vi "pH电极校准.vi"() -> ()   [LabVIEW 2016, in "斯坦道多参数.lvlib"]
uses:
  <vilib>/Utility/miscctls.llb/LVPointTypeDef.ctl
  <vilib>/Analysis/NI_AALBase.lvlib
panel:
  in  "校准停止":bool
  in  "校准启动":bool
  out "第二点校准值":dbl
  out "第一点校准值":dbl
  out "提示":string
  in  "校准模式":enum16{"两点校准", "单点校准"}(ring)
  out "最小值":sgl format="%.2g"
  out "最大值":sgl format="%.2g"
  out "变异系数":dbl format="%.6g"
  out "standard deviation":dbl caption="标准差" format="%0.2f"
  out "mean":dbl caption="均值" format="%0.2f"
  out "波形图表":sgl(graph) caption="历史曲线"
  out "当前检测值":dbl format="%#.2g"
  out "标液2":dbl
  out "标液1":dbl
  out "当前信号值":dbl format="%#.2g"
  out "偏移值补偿":dbl format="%#.2g"
  out "电极斜率":dbl
  out "电极零点":dbl
  # "酸碱度电极设定"
  # "mV"
  # "mV"
  # "%"
  # "pH"
  # "请选择校准模式:"
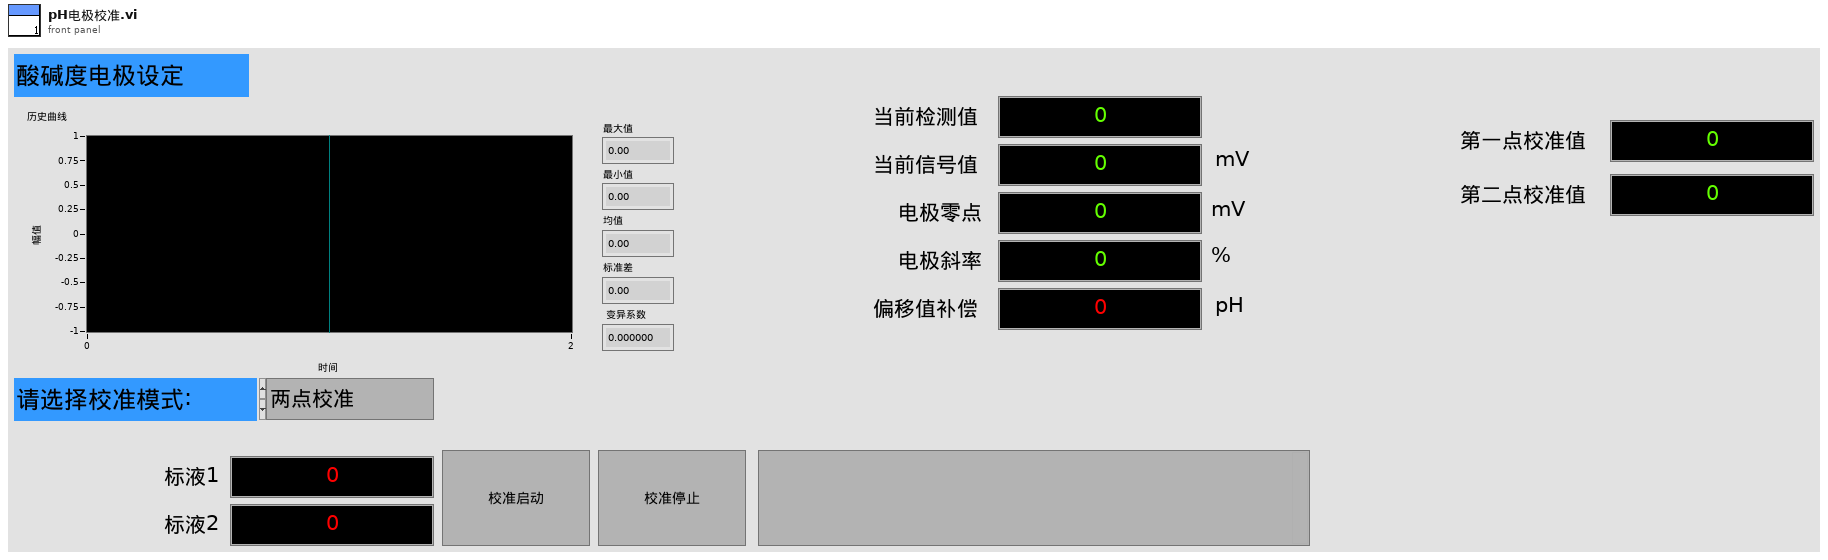
[diagram p1: front panel]
types:
  T1 = typedef "LVPointTypeDef.ctl" = cluster{"Horizontal":i16, "Vertical":i16}
  T2 = typedef "斯坦道多参数.lvlib/校准步骤.ctl" = enum16{"待机", "放置第一点标液", "第一点校准启动", "第一点校准写入", "第一点校准失败", "放置第二点标液", "第二点校准启动", "第二点校准写入", "第二点校准失败", "校准结果写入", "校准结束"}
  T3 = cluster{"电极状态标志":u16, "电极型号标志":u16, "酸碱度测量值":sgl, "温度测量值":sgl, "酸碱度信号值":sgl, "温度信号值":sgl, "酸碱度偏移修正值":sgl, "温度偏移修正值":sgl, "手动温度补偿值":sgl, "酸碱度电极零点":sgl, "酸碱度电极斜率":sgl, "第1点标准值记录":sgl, "第1点信号值记录":sgl, "第1点温度值记录":sgl, "第2点标准值记录":sgl, "第2点信号值记录":sgl, "第2点温度值记录":sgl, "命令滤波设定":u16, "温度模式":enum16{"ATC", "MTC"}, "生产批次":u16, "电极序号":u16, "串口地址":u16, "串口波特率":enum16{"9600", "19200", "115200"}, "串口校验位":enum16{"NONE", "ODD", "EVEN"}, "串口停止位":enum16{"1bit", "2bit"}, "第一点标准值":sgl, "第二点标准值":sgl}
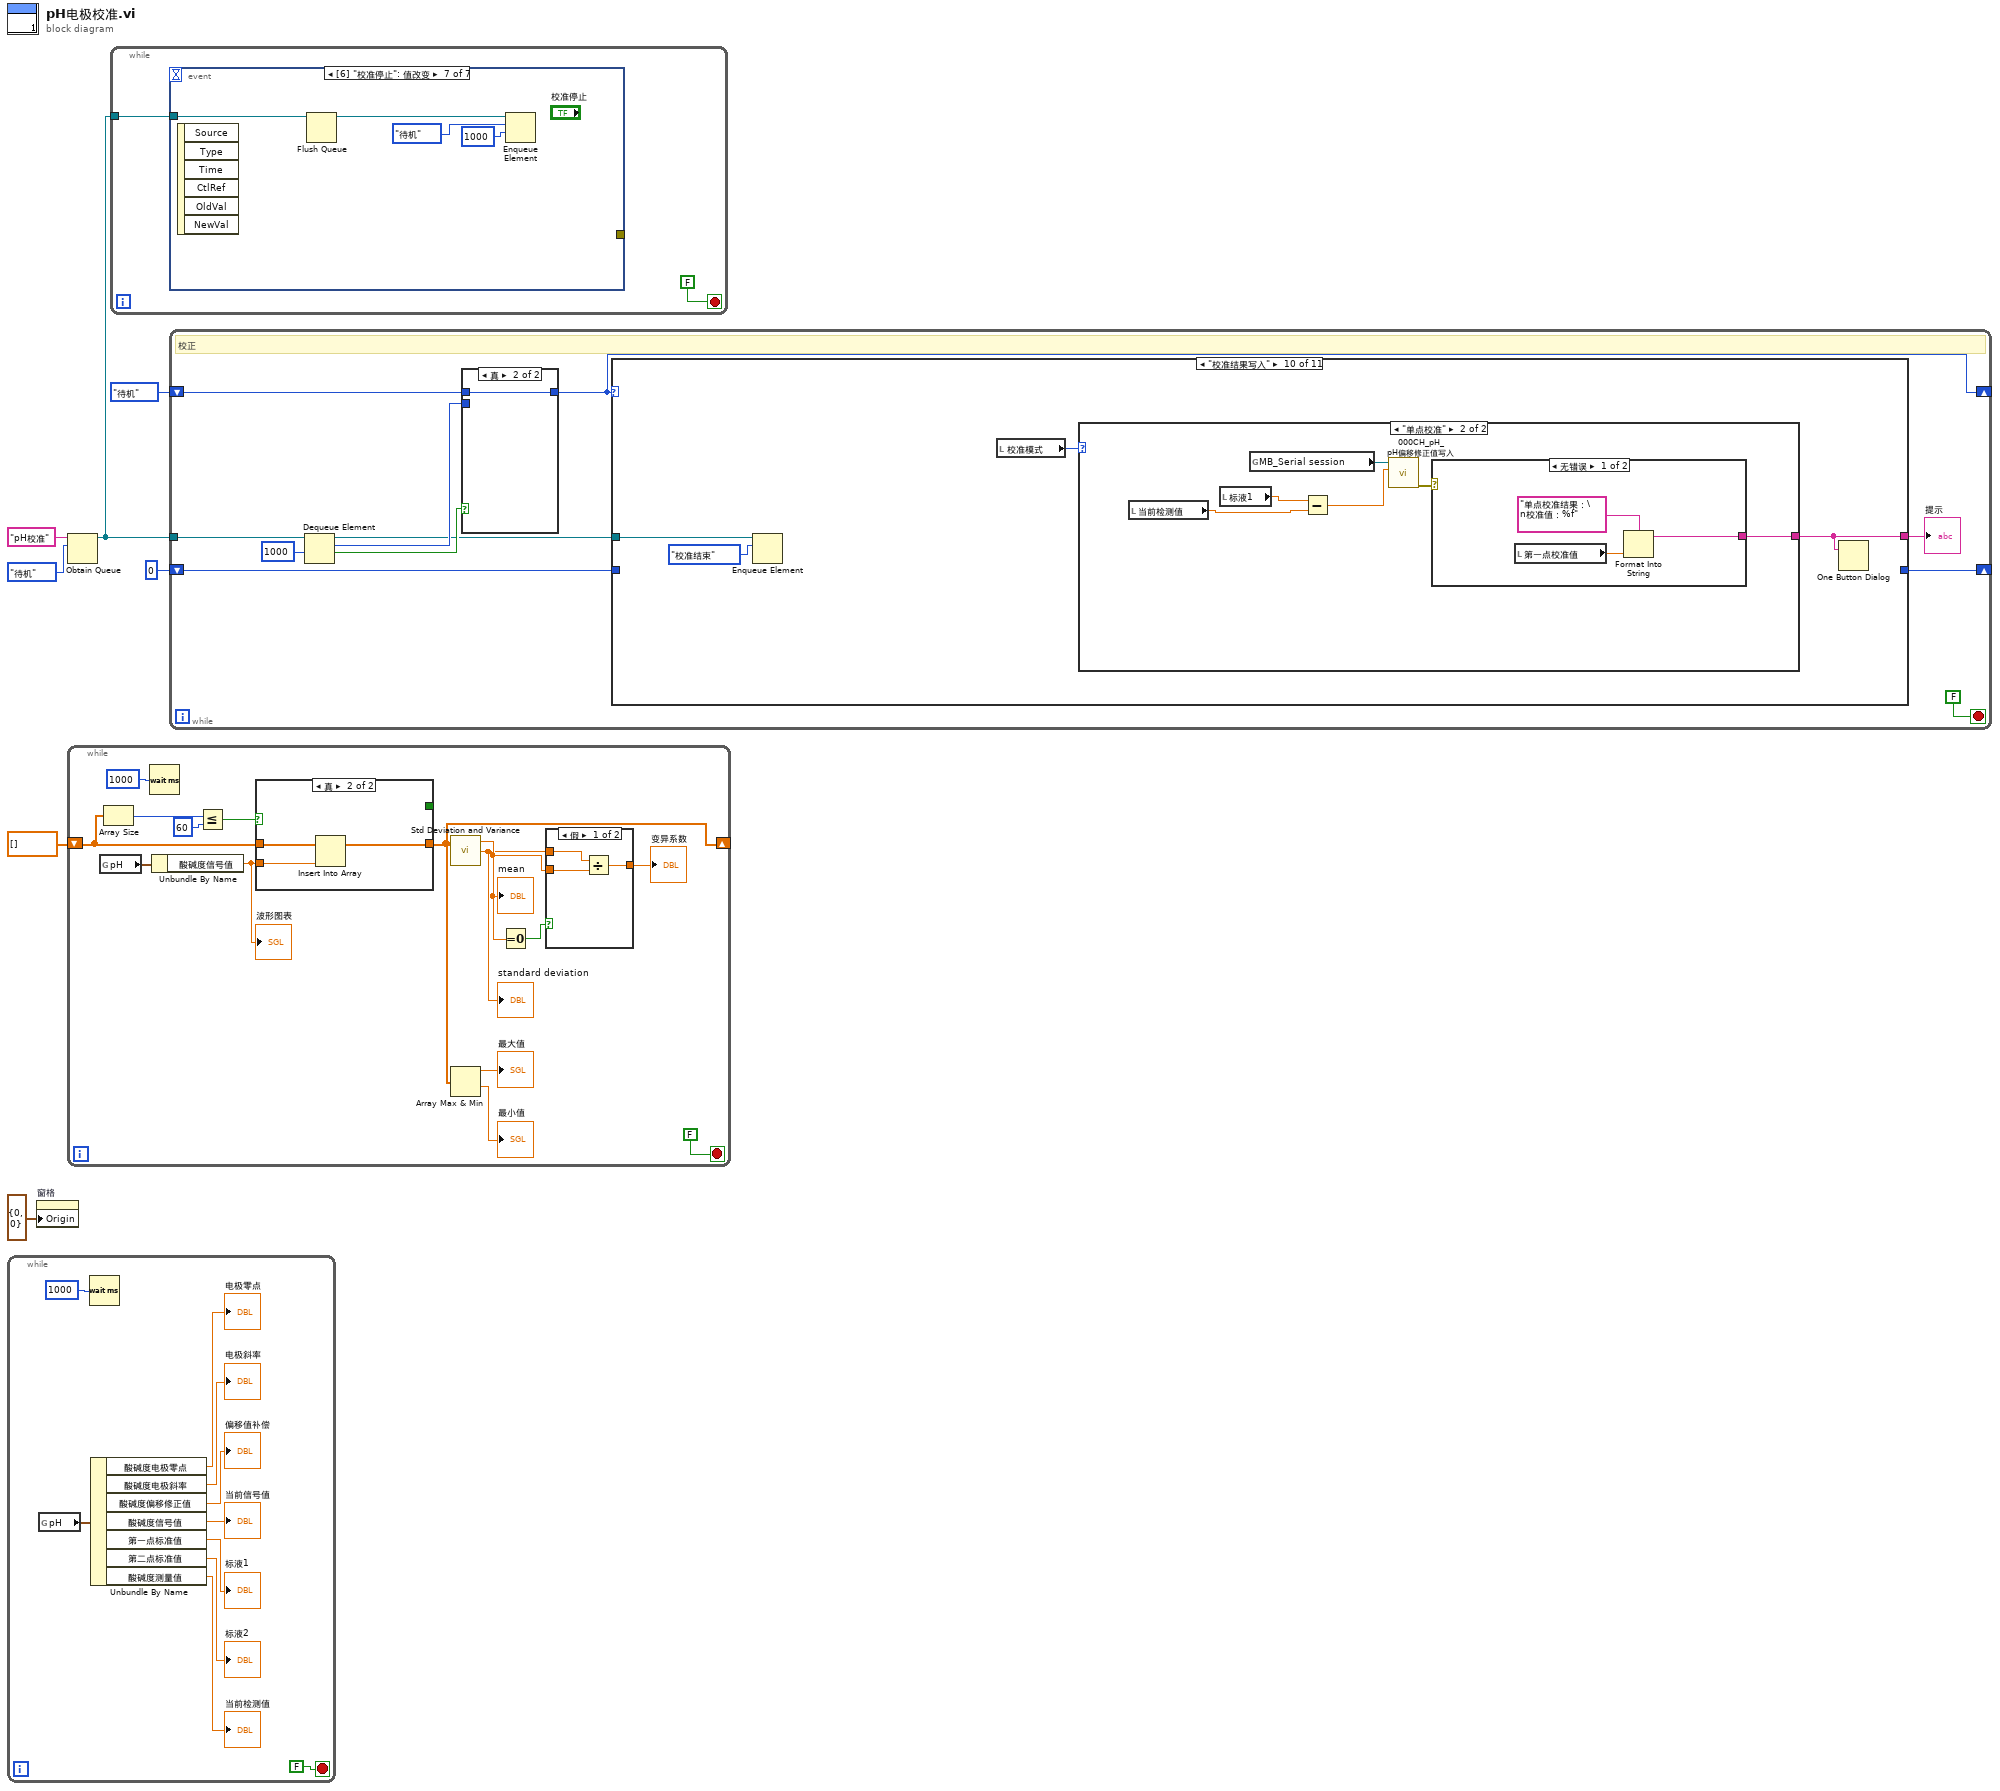
[diagram p0: block diagram]
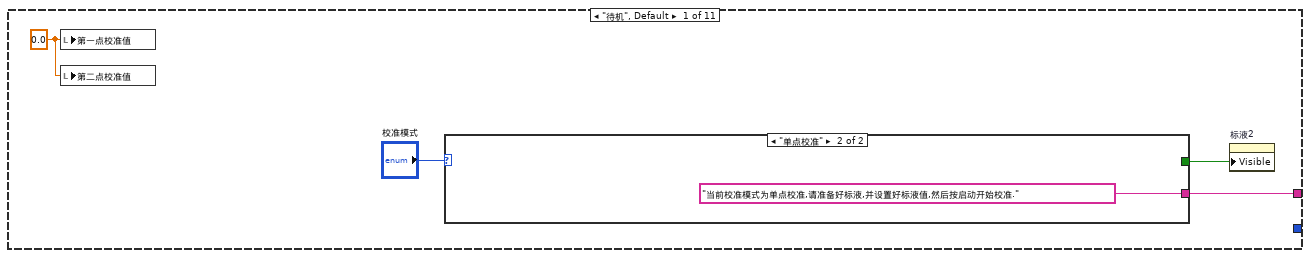
[diagram p3: hidden frame]
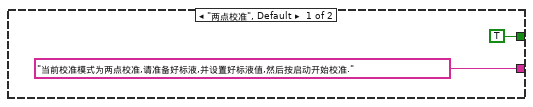
[diagram p4: hidden frame]
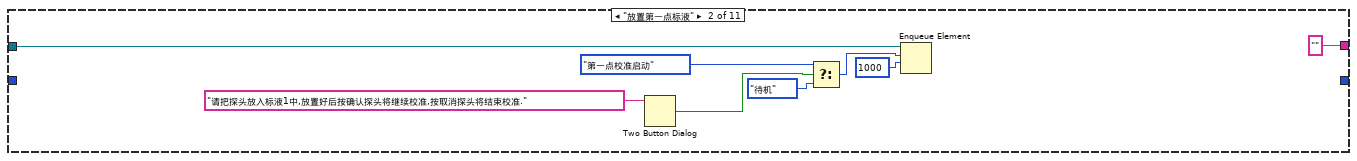
[diagram p5: hidden frame]
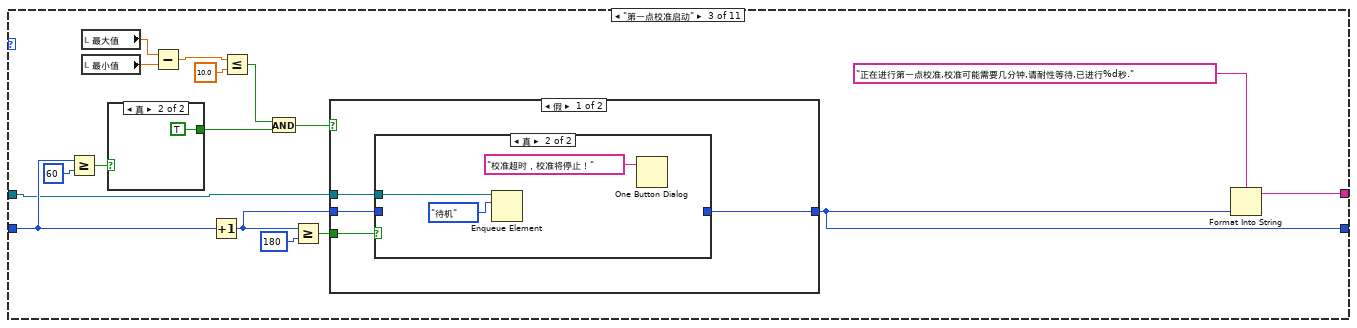
[diagram p6: hidden frame]
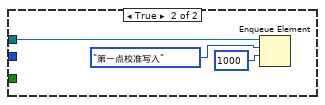
[diagram p8: hidden frame]
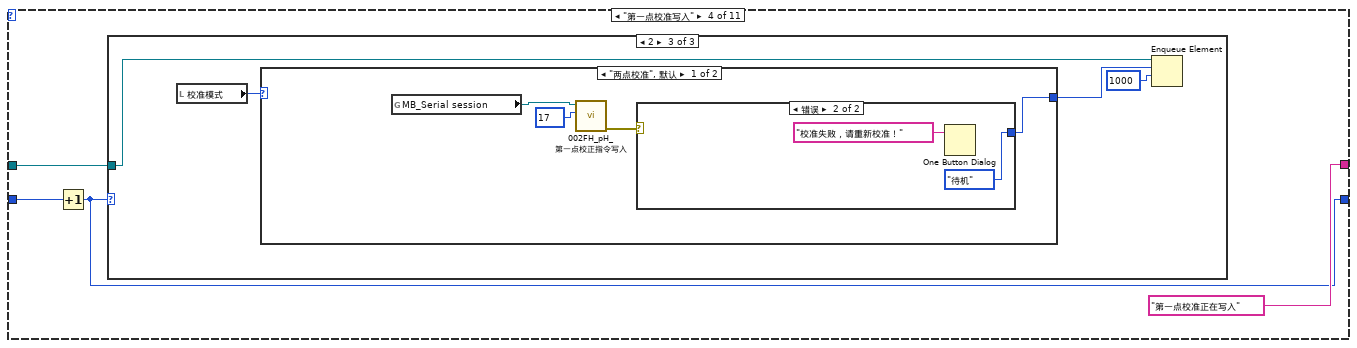
[diagram p10: hidden frame]
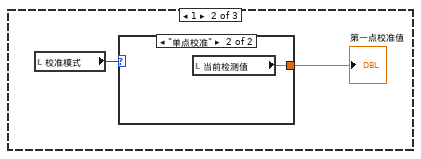
[diagram p12: hidden frame]
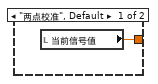
[diagram p13: hidden frame]
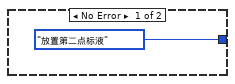
[diagram p14: hidden frame]
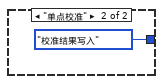
[diagram p15: hidden frame]
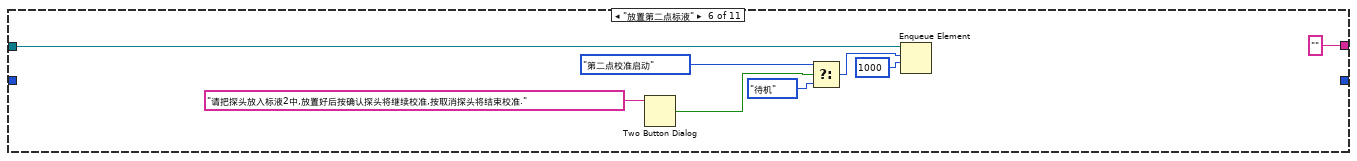
[diagram p17: hidden frame]
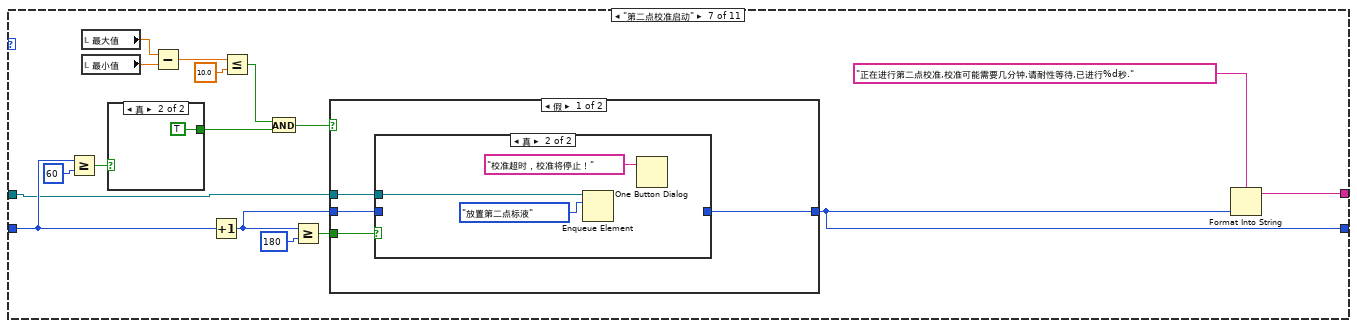
[diagram p18: hidden frame]
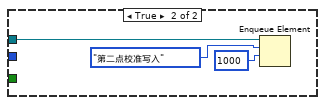
[diagram p20: hidden frame]
diagram:
  n1 = while {
    stop <- FALSE stop-if-true
    n2 = global read "国弘过程全局变量.vi" "pH"() -> (w15:T3)
    n3 = Wait (ms)(milliseconds to wait=u32 1000 ("等待时间（毫秒）")) -> ()  [unwired: 1 out]
    n4 = Unbundle By Name(w15) -> ("酸碱度电极零点"=→"电极零点":sgl, "酸碱度电极斜率"=→"电极斜率":sgl, "酸碱度偏移修正值"=→"偏移值补偿":sgl, "酸碱度信号值"=→"当前信号值":sgl, "第一点标准值"=→"标液1":sgl, "第二点标准值"=→"标液2":sgl, "酸碱度测量值"=→"当前检测值":sgl)
  }
  n5 = property on="窗格" class="Pane"("Origin"=T1 {"Horizontal"=0, "Vertical"=0} ("原点")) -> ()  [unwired: 2 in, 2 out]
  n6 = Obtain Queue(name (unnamed)="pH校准" ("名称（未命名）"), element data type=校准步骤."待机" ("枚举")) -> (queue out=w2:refnum<queue>)  [unwired: 3 in, 2 out]
  n7 = while {
    shift-right: [w24] -> _
    shift-left: sgl[] [] -> [w28]
    stop <- FALSE stop-if-true
    n8 = global read "国弘过程全局变量.vi" "pH"() -> (w25:T3)
    n9 = Array Size(array=w28) -> (size(s)=w30:i32)
    n10 = Wait (ms)(milliseconds to wait=u32 1000 ("等待时间（毫秒）")) -> ()  [unwired: 1 out]
    n11 = Unbundle By Name(w25) -> ("酸碱度信号值"=w18:sgl)
    "波形图表" <- w18
    n12 = Less Or Equal?(x=w30, y=60) -> (x <= y?=w29:bool)
    n13 = case shown="真" w29 {
      tunnel: w28 -> [w41 w44]
      tunnel: w18 -> [w39 w43]
      tunnel: [w37 w42] -> w24
      tunnel: [TRUE _] -> _
      frame False {
        n14 = Replace Array Subset(array=w41, new element=w39) -> (w40:sgl[])  [unwired: 1 in]
        n15 = Rotate 1D Array(1:w40, 2:-1 ("n")) -> (0:w37:sgl[])
      }
      frame True {
        n16 = Insert Into Array(array=w44, new element=w43) -> (w42:sgl[])  [unwired: 1 in]
      }
    }
    n17 = call <vilib>:"Std Deviation and Variance.vi"("X"=w24) -> ("mean"=w20:dbl, "standard deviation"=w19:dbl)  [unwired: 1 in, 1 out]
    "mean" <- w20
    "standard deviation" <- w19
    n18 = Array Max & Min(array=w24) -> (max value=→"最大值":sgl, min value=→"最小值":sgl)  [unwired: 2 out]
    n19 = Equal To 0?(x=w20) -> (x = 0?=w27:bool)
    n20 = case shown="假" w27 {
      tunnel: w19 -> [w35 _]
      tunnel: [w34 _] -> w21
      tunnel: w20 -> [w33 _]
      frame False {
        n21 = Divide(x=w35, y=w33) -> (x/y=w34:dbl)
      }
      frame True {
      }
    }
    "变异系数" <- w21
  }
  n22 = while {
    tunnel: w2 -> [w45]
    stop <- FALSE stop-if-true
    n23 = event shown="[6] \"校准停止\": 值改变" {
      selector: _ -> [_ _ _ _ _ _ _]
      dyn-events: _ -> [_ _ _ _ _ _ _]
      timeout: _ -> [_ _ _ _ _ _ _]
      tunnel: [_ _ w52 w55 w58 _ _] -> _
      tunnel: w45 -> [_ _ _ _ _ w60 w62]
      event Timeout {
        n24 = event-data() -> ()  [unwired: 1 in, 3 out]
      }
      event "标液1", "标液2", "偏移值补偿": Mouse Down {
        n25 = event-data() -> ("CtlRef"=w50:refnum<vi>)  [unwired: 1 in, 7 out]
        n26 = property class="DigNum (严格)"(reference=w50) -> (reference out=w47:refnum<vi>, "Value"=w48:dbl)  [unwired: 1 in, 1 out]
        n27 = call "数字键盘.vi"("OldNumber"=w48) -> ("NewNumber"=w49:sgl)
        n28 = property class="DigNum (严格)"(reference=w47, "Val(Sgnl)"=w49) -> ()  [unwired: 1 in, 2 out]
      }
      event "偏移值补偿": Value Change {
        n29 = event-data() -> ("NewVal"=w53:dbl)  [unwired: 1 in, 5 out]
        n30 = global read "多参数全局变量.vi" "MB_Serial session"() -> (w51:refnum<class "MB_Master_Serial.lvclass">)
        n31 = call "000CH_pH_pH偏移修正值写入.vi"("数值"=w53, "MB_Serial session in"=w51) -> ("error out"=w52:errorcluster)  [unwired: 8 in, 1 out]
      }
      event "标液1": Value Change {
        n32 = event-data() -> ("NewVal"=w56:dbl)  [unwired: 1 in, 5 out]
        n33 = global read "多参数全局变量.vi" "MB_Serial session"() -> (w54:refnum<class "MB_Master_Serial.lvclass">)
        n34 = call "0030H_pH_第一点标准值写入.vi"("数值"=w56, "MB_Serial session in"=w54) -> ("error out"=w55:errorcluster)  [unwired: 8 in, 1 out]
      }
      event "标液2": Value Change {
        n35 = event-data() -> ("NewVal"=w59:dbl)  [unwired: 1 in, 5 out]
        n36 = global read "多参数全局变量.vi" "MB_Serial session"() -> (w57:refnum<class "MB_Master_Serial.lvclass">)
        n37 = call "0033H_pH_第二点标准值写入.vi"("数值"=w59, "MB_Serial session in"=w57) -> ("error out"=w58:errorcluster)  [unwired: 8 in, 1 out]
      }
      event "校准启动": Value Change {
        n38 = event-data() -> ()  [unwired: 1 in, 6 out]
        n39 = Enqueue Element(queue=w60, element=校准步骤."放置第一点标液" ("元素")) -> ()  [unwired: 2 in, 3 out]
      }
      event "校准停止": Value Change {
        n40 = event-data() -> ()  [unwired: 1 in, 6 out]
        n41 = Flush Queue(queue=w62) -> (queue out=w63:refnum<queue>)  [unwired: 1 in, 2 out]
        n42 = Enqueue Element(queue=w63, element=校准步骤."待机" ("元素"), timeout in ms (-1)=1000 ("超时毫秒(-1)")) -> ()  [unwired: 1 in, 3 out]
      }
    }
  }
  n43 = while "While循环" {
    shift-right: [w67] -> _
    shift-left: 校准步骤."待机" ("枚举") -> [w68]
    shift-right: [w74] -> _
    shift-left: 0 -> [w75]
    tunnel: w2 -> [w72]
    stop <- FALSE stop-if-true
    # "校正"
    n44 = Dequeue Element(queue=w72, timeout in ms (-1)=1000 ("超时毫秒(-1)")) -> (queue out=w66:refnum<queue>, element=w69:T2, timed out?=w70:bool)  [unwired: 1 in, 1 out]
    n45 = case shown="真" w70 {
      tunnel: w69 -> [w77 _]
      tunnel: [w77 w78] -> w67
      tunnel: w68 -> [_ w78]
      frame False {
      }
      frame True {
      }
    }
    n46 = case shown="\"校准结果写入\"" w67 {
      tunnel: [w82 "" ("提示") w109 "第一点校准正在写入" ("提示") _ "" ("提示") w166 "第二点校准正在写入" ("提示") _ w197 w225] -> w73
      tunnel: w75 -> [_ _ w103 w125 _ _ w160 w182 _ _ _]
      tunnel: [_ _ w94 w124 _ _ w151 w181 _ _ _] -> w74
      tunnel: w66 -> [_ w92 w97 w123 _ w149 w154 w180 _ w196 _]
      frame "待机", Default {
        w79 = 0.0 ("第一点校准值")
        n47 = local write "第一点校准值"(w79) -> ()
        n48 = local write "第二点校准值"(w79) -> ()
        n49 = case shown="\"单点校准\"" "校准模式" {
          tunnel: ["当前校准模式为两点校准,请准备好标液,并设置好标液值,然后按启动开始校准." ("提示") "当前校准模式为单点校准,请准备好标液,并设置好标液值,然后按启动开始校准." ("提示")] -> w82
          tunnel: [TRUE ("可见") _] -> w81
          frame "两点校准", Default {
          }
          frame "单点校准" {
          }
        }
        n50 = property on="标液2" class="DigNum (严格)"("Visible"=w81) -> ()  [unwired: 2 in, 2 out]
      }
      frame "放置第一点标液" {
        n51 = Two Button Dialog(message="请把探头放入标液1中,放置好后按确认探头将继续校准,按取消探头将结束校准." ("消息")) -> (T button?=w90:bool)  [unwired: 2 in]
        n52 = Select(t=校准步骤."第一点校准启动" ("元素"), s=w90, f=校准步骤."待机" ("元素")) -> (s? t:f=w87:T2)
        n53 = Enqueue Element(queue=w92, element=w87, timeout in ms (-1)=1000 ("超时毫秒(-1)")) -> ()  [unwired: 1 in, 3 out]
      }
      frame "第一点校准启动" {
        n54 = Greater Or Equal?(x=w103, y=60) -> (x >= y?=w104:bool)
        n55 = local read "最大值"() -> (w100:sgl)
        n56 = local read "最小值"() -> (w101:sgl)
        n57 = case shown="真" w104 {
          tunnel: [_ TRUE] -> w102
          frame False {
          }
          frame True {
          }
        }
        n58 = Subtract(x=w100, y=w101) -> (x-y=w99:sgl)
        n59 = Increment(x=w103) -> (x+1=w95:i32)
        n60 = Less Or Equal?(x=w99, y=10.0) -> (x <= y?=w107:bool)
        n61 = And(x=w107, y=w102) -> (x .and. y?=w98:bool)
        n62 = Greater Or Equal?(x=w95, y=180) -> (x >= y?=w96:bool)
        n63 = case shown="假" w98 {
          tunnel: w97 -> [w113 w121]
          tunnel: w96 -> [w114 _]
          tunnel: w95 -> [w112 _]
          tunnel: [w111 _] -> w94
          frame False {
            n64 = case shown="真" w114 {
              tunnel: w113 -> [_ w118]
              tunnel: w112 -> [w115 _]
              tunnel: [w115 _] -> w111
              frame False {
              }
              frame True {
                n65 = Enqueue Element(queue=w118, element=校准步骤."待机" ("元素")) -> ()  [unwired: 2 in, 3 out]
                n66 = One Button Dialog(message="校准超时，校准将停止！" ("消息")) -> ()  [unwired: 1 in, 1 out]
              }
            }
          }
          frame True {
            n67 = Enqueue Element(queue=w121, element=校准步骤."第一点校准写入" ("元素"), timeout in ms (-1)=1000 ("超时毫秒(-1)")) -> ()  [unwired: 1 in, 3 out]
          }
        }
        n68 = Format Into String(format string="正在进行第一点校准,校准可能需要几分钟,请耐性等待,已进行%d秒." ("格式字符串"), w94) -> (resulting string=w109:string)  [unwired: 2 in, 1 out]
      }
      frame "第一点校准写入" {
        n69 = Increment(x=w125) -> (x+1=w124:i32)
        n70 = case shown="2" w124 {
          tunnel: w123 -> [_ _ w134]
          frame 0, Default {
          }
          frame 1 {
            n71 = local read "校准模式"() -> (w127:enum16{"两点校准", "单点校准"})
            n72 = case shown="\"单点校准\"" w127 {
              tunnel: [w129 w130] -> w128
              frame "两点校准", Default {
                n73 = local read "当前信号值"() -> (w129:dbl)
              }
              frame "单点校准" {
                n74 = local read "当前检测值"() -> (w130:dbl)
              }
            }
            "第一点校准值" <- w128
          }
          frame 2 {
            n75 = local read "校准模式"() -> (w133:enum16{"两点校准", "单点校准"})
            n76 = case shown="\"两点校准\", 默认" w133 {
              tunnel: [w138 校准步骤."校准结果写入" ("元素")] -> w132
              frame "两点校准", Default {
                n77 = global read "多参数全局变量.vi" "MB_Serial session"() -> (w137:refnum<class "MB_Master_Serial.lvclass">)
                n78 = call "002FH_pH_第一点校正指令写入.vi"("数值"=u16 17, "MB_Serial session in"=w137) -> ("error out"=w135:errorcluster)  [unwired: 8 in, 1 out]
                n79 = case shown="错误" w135 {
                  tunnel: [校准步骤."放置第二点标液" ("元素") 校准步骤."待机" ("元素")] -> w138
                  frame No Error {
                  }
                  frame Error {
                    n80 = One Button Dialog(message="校准失败，请重新校准！" ("消息")) -> ()  [unwired: 1 in, 1 out]
                  }
                }
              }
              frame "单点校准" {
              }
            }
            n81 = Enqueue Element(queue=w134, element=w132, timeout in ms (-1)=1000 ("超时毫秒(-1)")) -> ()  [unwired: 1 in, 3 out]
          }
        }
      }
      frame "第一点校准失败" {
      }
      frame "放置第二点标液" {
        n82 = Two Button Dialog(message="请把探头放入标液2中,放置好后按确认探头将继续校准,按取消探头将结束校准." ("消息")) -> (T button?=w147:bool)  [unwired: 2 in]
        n83 = Select(t=校准步骤."第二点校准启动" ("元素"), s=w147, f=校准步骤."待机" ("元素")) -> (s? t:f=w144:T2)
        n84 = Enqueue Element(queue=w149, element=w144, timeout in ms (-1)=1000 ("超时毫秒(-1)")) -> ()  [unwired: 1 in, 3 out]
      }
      frame "第二点校准启动" {
        n85 = Greater Or Equal?(x=w160, y=60) -> (x >= y?=w161:bool)
        n86 = local read "最大值"() -> (w157:sgl)
        n87 = local read "最小值"() -> (w158:sgl)
        n88 = case shown="真" w161 {
          tunnel: [_ TRUE] -> w159
          frame False {
          }
          frame True {
          }
        }
        n89 = Subtract(x=w157, y=w158) -> (x-y=w156:sgl)
        n90 = Increment(x=w160) -> (x+1=w152:i32)
        n91 = Less Or Equal?(x=w156, y=10.0) -> (x <= y?=w164:bool)
        n92 = And(x=w164, y=w159) -> (x .and. y?=w155:bool)
        n93 = Greater Or Equal?(x=w152, y=180) -> (x >= y?=w153:bool)
        n94 = case shown="假" w155 {
          tunnel: w154 -> [w170 w178]
          tunnel: w153 -> [w171 _]
          tunnel: w152 -> [w169 _]
          tunnel: [w168 _] -> w151
          frame False {
            n95 = case shown="真" w171 {
              tunnel: w170 -> [_ w175]
              tunnel: w169 -> [w172 _]
              tunnel: [w172 _] -> w168
              frame False {
              }
              frame True {
                n96 = Enqueue Element(queue=w175, element=校准步骤."放置第二点标液" ("元素")) -> ()  [unwired: 2 in, 3 out]
                n97 = One Button Dialog(message="校准超时，校准将停止！" ("消息")) -> ()  [unwired: 1 in, 1 out]
              }
            }
          }
          frame True {
            n98 = Enqueue Element(queue=w178, element=校准步骤."第二点校准写入" ("元素"), timeout in ms (-1)=1000 ("超时毫秒(-1)")) -> ()  [unwired: 1 in, 3 out]
          }
        }
        n99 = Format Into String(format string="正在进行第二点校准,校准可能需要几分钟,请耐性等待,已进行%d秒." ("格式字符串"), w151) -> (resulting string=w166:string)  [unwired: 2 in, 1 out]
      }
      frame "第二点校准写入" {
        n100 = Increment(x=w182) -> (x+1=w181:i32)
        n101 = case shown="2" w181 {
          tunnel: w180 -> [_ _ w190]
          frame 0, Default {
          }
          frame 1 {
            n102 = local read "当前信号值"() -> (→"第二点校准值":dbl)
          }
          frame 2 {
            n103 = global read "多参数全局变量.vi" "MB_Serial session"() -> (w187:refnum<class "MB_Master_Serial.lvclass">)
            n104 = call "0032H_pH_第二点校正指令写入.vi"("数值"=u16 33, "MB_Serial session in"=w187) -> ("error out"=w186:errorcluster)  [unwired: 8 in, 1 out]
            n105 = case shown="错误" w186 {
              tunnel: [校准步骤."校准结果写入" ("元素") 校准步骤."放置第二点标液" ("元素")] -> w185
              frame No Error {
              }
              frame Error {
                n106 = One Button Dialog(message="校准失败，请重新校准！" ("消息")) -> ()  [unwired: 1 in, 1 out]
              }
            }
            n107 = Enqueue Element(queue=w190, element=w185, timeout in ms (-1)=1000 ("超时毫秒(-1)")) -> ()  [unwired: 1 in, 3 out]
          }
        }
      }
      frame "第二点校准失败" {
      }
      frame "校准结果写入" {
        n108 = Enqueue Element(queue=w196, element=校准步骤."校准结束" ("元素")) -> ()  [unwired: 2 in, 3 out]
        n109 = local read "校准模式"() -> (w194:enum16{"两点校准", "单点校准"})
        n110 = case shown="\"单点校准\"" w194 {
          tunnel: [w200 w219] -> w197
          frame "两点校准", Default {
            (unwired) u16 0 items=["OK", "第一点校正通过", "第二点校正通过", "校正失败,电极零点超出范围", "校正失败,电极斜率超出范围", "第三点校正通过"] ("电极状态标志")
            n111 = global read "国弘过程全局变量.vi" "pH"() -> (w199:T3)
            n112 = Unbundle By Name(w199) -> ("电极状态标志"=w198:u16)
            n113 = case shown="0, 默认" w198 {
              selector: w198 -> [w202 _ w211]
              tunnel: [w201 w206 w210] -> w200
              frame 0, Default {
                n114 = case shown="0, 默认" w202 {
                  tunnel: ["校正未正常启动，请重新校正" "第一点校准通过" "第二点校准通过"] -> w201
                  frame 0, Default {
                  }
                  frame 1 {
                  }
                  frame 2 {
                  }
                }
              }
              frame 2 {
                n115 = local read "第一点校准值"() -> (w208:dbl)
                n116 = local read "第二点校准值"() -> (w209:dbl)
                n117 = Format Into String(format string="两点校准结果：\n第一点校准值：%f\n第二点校准值：%f" ("提示"), w208, w209) -> (resulting string=w206:string)  [unwired: 2 in, 1 out]
              }
              frame 3, 4 {
                n118 = case shown="4" w211 {
                  tunnel: ["校正失败，电极零点超出范围" "校正失败，电极斜率超出范围"] -> w210
                  frame 3, Default {
                  }
                  frame 4 {
                  }
                }
              }
            }
          }
          frame "单点校准" {
            n119 = local read "当前检测值"() -> (w218:dbl)
            n120 = local read "标液1"() -> (w217:dbl)
            n121 = global read "多参数全局变量.vi" "MB_Serial session"() -> (w216:refnum<class "MB_Master_Serial.lvclass">)
            n122 = Subtract(x=w217, y=w218) -> (x-y=w214:dbl)
            n123 = call "000CH_pH_pH偏移修正值写入.vi"("数值"=w214, "MB_Serial session in"=w216) -> ("error out"=w215:errorcluster)  [unwired: 8 in, 1 out]
            n124 = case shown="无错误" w215 {
              tunnel: [w220 "校准失败"] -> w219
              frame No Error {
                n125 = local read "第一点校准值"() -> (w222:dbl)
                n126 = Format Into String(format string="单点校准结果：\n校准值：%f" ("提示"), w222) -> (resulting string=w220:string)  [unwired: 2 in, 1 out]
              }
              frame Error {
                n127 = One Button Dialog(message="校准失败，请重新校准！" ("消息")) -> ()  [unwired: 1 in, 1 out]
              }
            }
          }
        }
        n128 = One Button Dialog(message=w197) -> ()  [unwired: 1 in, 1 out]
      }
      frame "校准结束" {
        n129 = local read "提示"() -> (w225:string)
      }
    }
    "提示" <- w73
  }
